vi "Origin_Export_7_27a_JW.vi"(6 "Input Conditions":T1, 7 "Analysis Array":string[][](array[string]), 8 "error in (no error)":errorcluster, 9 "Parameter Worksheet Name":string, 10 "Parameter Folder Script":string, 11 "Origin.IOApplication":refnum<k7>) -> (0 "error out":errorcluster, 2 "Origin.Worksheet":refnum<k7>, 3 "reference out":refnum<k7>)   [LabVIEW 2012]
panel:
  out "Dep Active Window":string
  out "Indep Unit":string
  out "Dep Unit":string
  out "Dep Used":string
  out "Indep Used":string
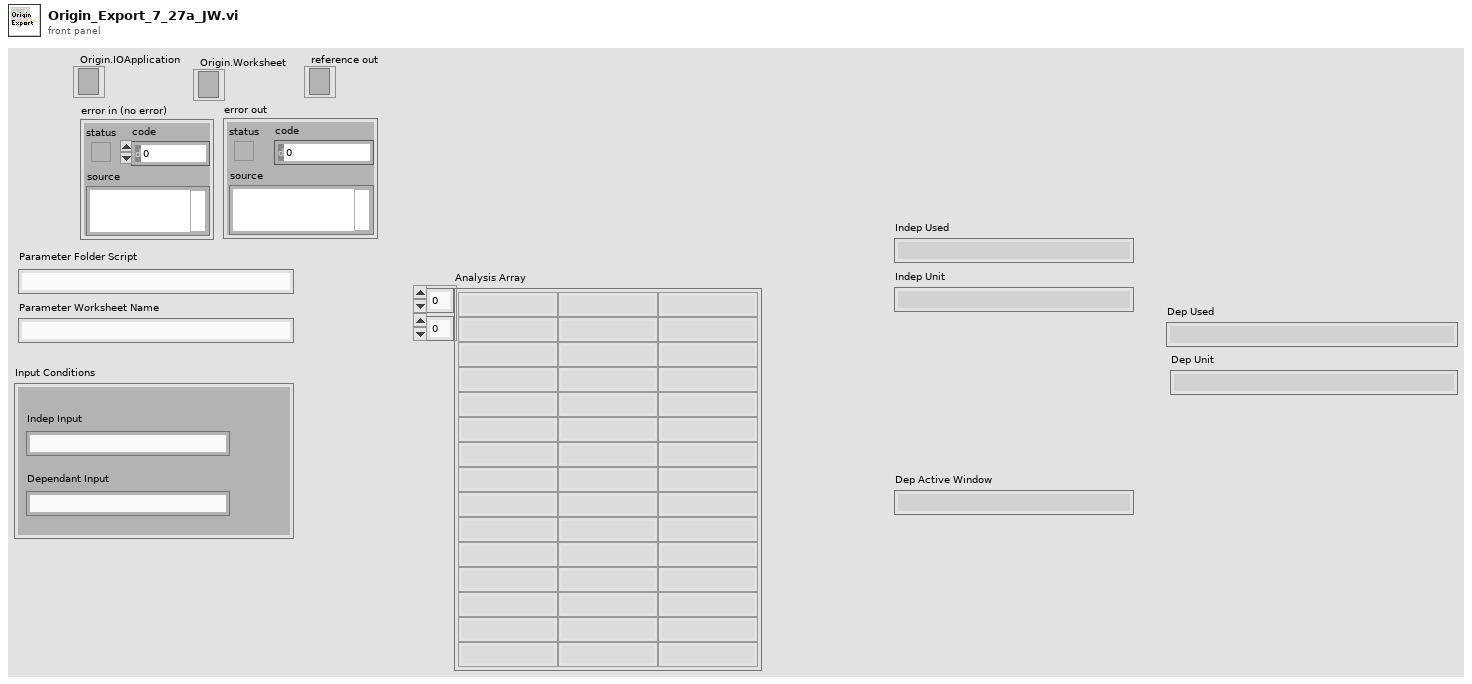
[diagram p1: front panel]
types:
  T1 = cluster{"Indep Input":string, "Dependant Input":string}
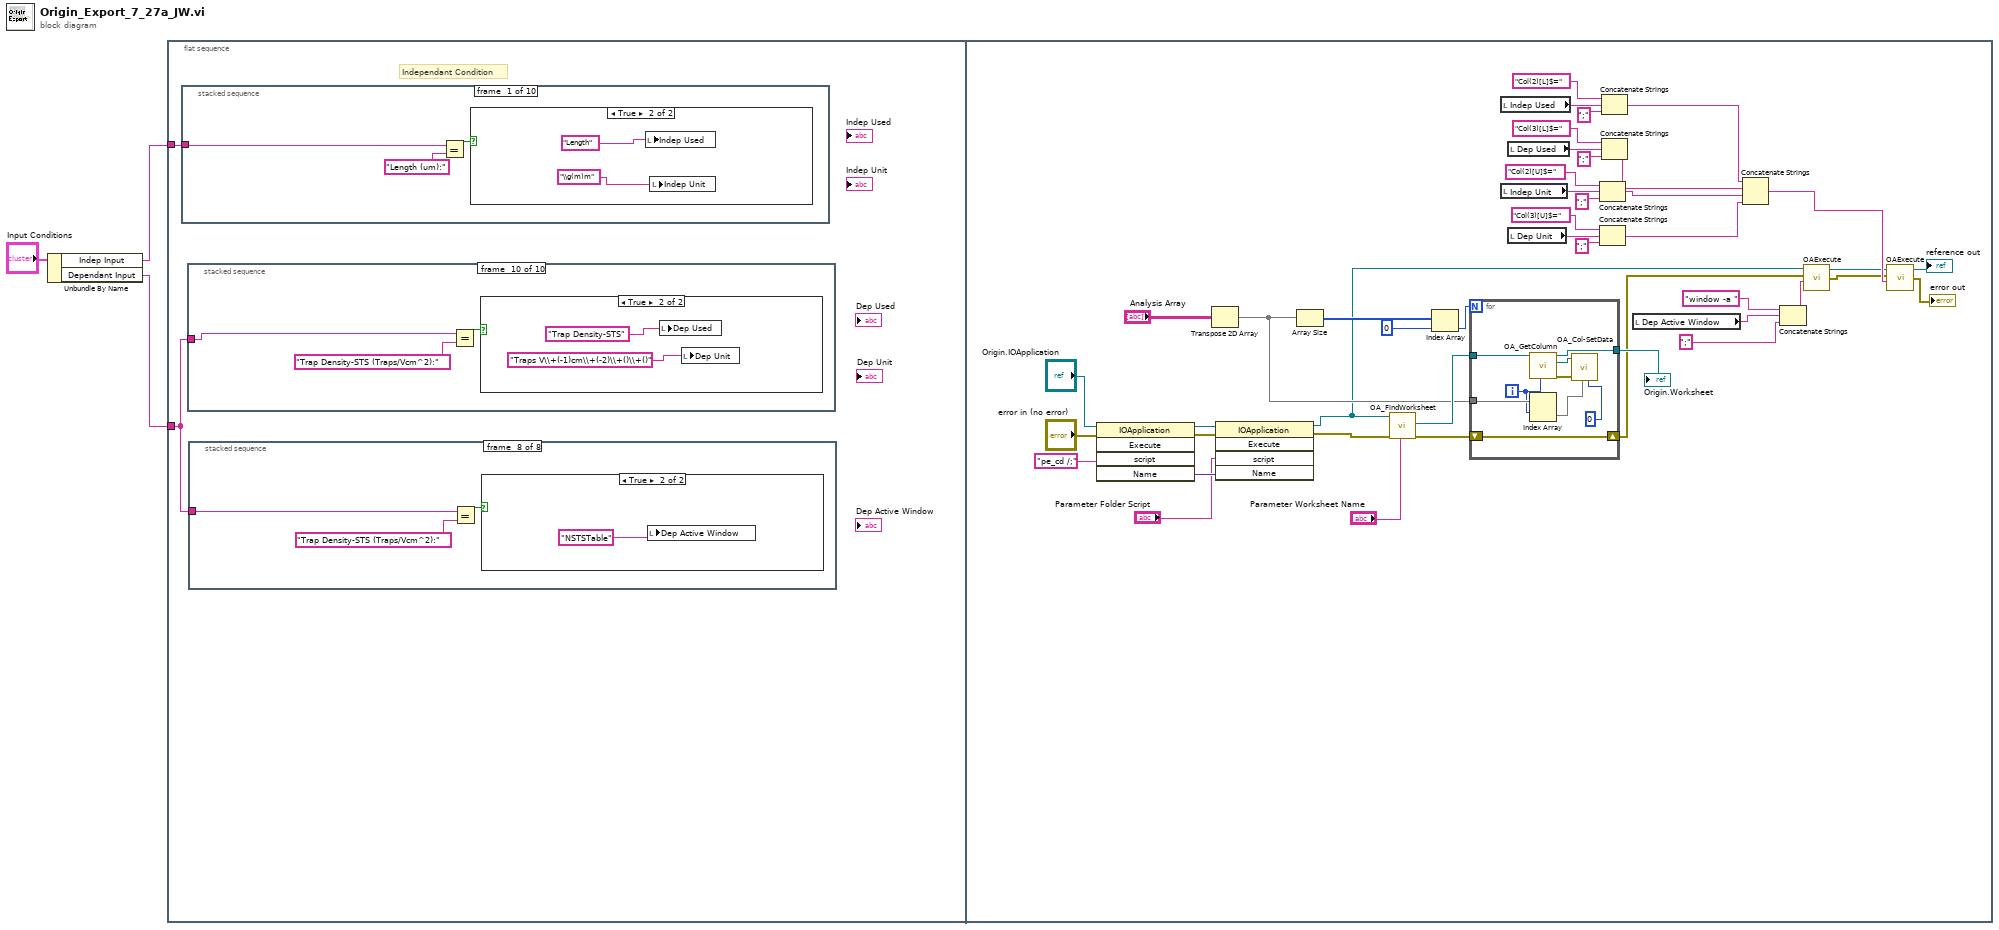
[diagram p0: block diagram]
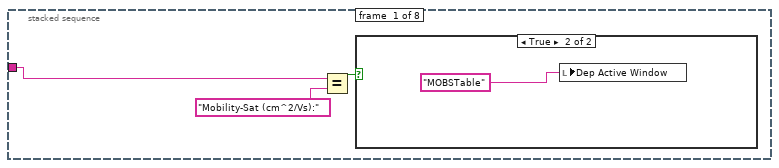
[diagram p2: hidden frame]
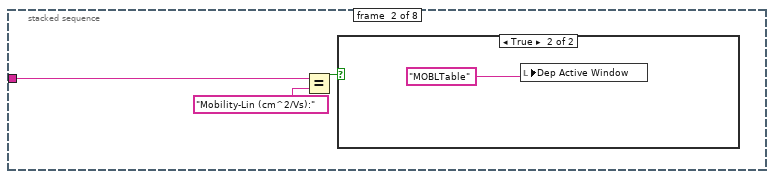
[diagram p4: hidden frame]
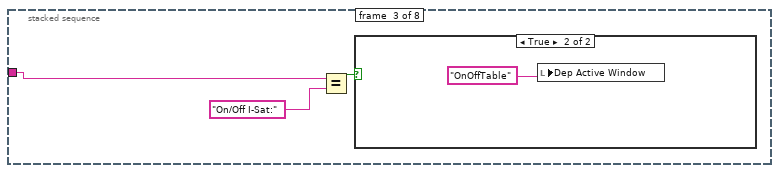
[diagram p6: hidden frame]
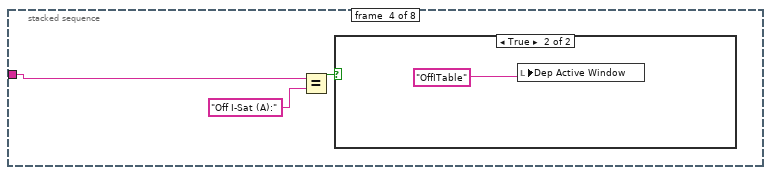
[diagram p8: hidden frame]
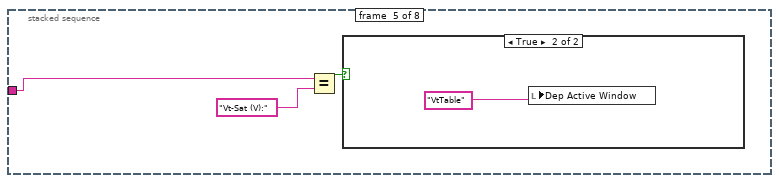
[diagram p10: hidden frame]
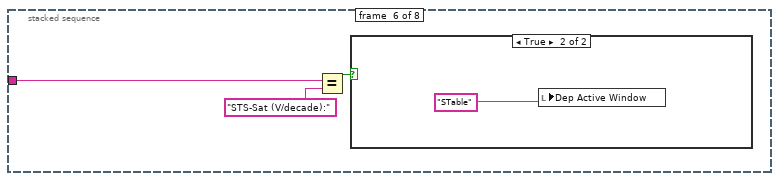
[diagram p12: hidden frame]
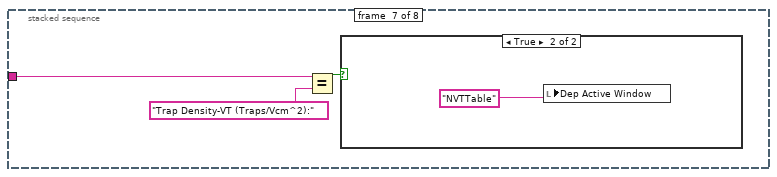
[diagram p14: hidden frame]
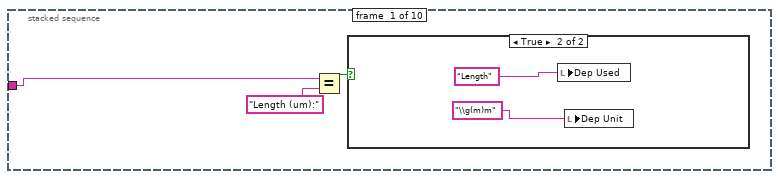
[diagram p17: hidden frame]
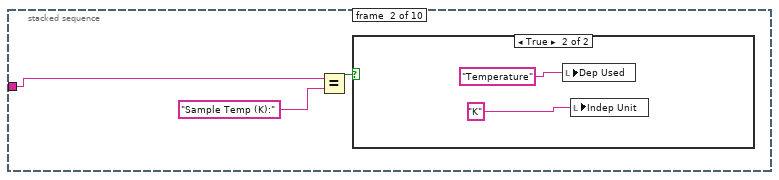
[diagram p19: hidden frame]
diagram:
  n1 = Unbundle By Name("Input Conditions") -> ("Indep Input"=w2:string, "Dependant Input"=w1:string)
  n2 = flat-sequence {
    tunnel: w2 -> [w5]
    tunnel: w1 -> [w4]
    frame #0 {
      # "Independant Condition"
      n3 = stacked-sequence {
        tunnel: w5 -> [w88 w93 w98 w103 w108 w113 w118 w123 w128 w133]
        frame #0 {
          n4 = Equal?(x=w88, y="Length (um):") -> (x = y?=w89:bool)
          n5 = case shown="True" w89 {
            frame False {
            }
            frame True {
              n6 = local write "Indep Used"("Length") -> ()
              n7 = local write "Indep Unit"("\\g(m)m") -> ()
            }
          }
        }
        frame #1 {
          n8 = Equal?(x=w93, y="Sample Temp (K):") -> (x = y?=w94:bool)
          n9 = case shown="True" w94 {
            frame False {
            }
            frame True {
              n10 = local write "Indep Used"("Temperature") -> ()
              n11 = local write "Indep Unit"("K") -> ()
            }
          }
        }
        frame #2 {
          n12 = Equal?(x=w98, y="Mobility-Sat (cm^2/Vs):") -> (x = y?=w99:bool)
          n13 = case shown="True" w99 {
            frame False {
            }
            frame True {
              n14 = local write "Indep Used"("Saturation Mobility") -> ()
              n15 = local write "Indep Unit"("cm\\+(2)V\\+(-1)s\\+(-1)") -> ()
            }
          }
        }
        frame #3 {
          n16 = Equal?(x=w103, y="Mobility-Lin (cm^2/Vs):") -> (x = y?=w104:bool)
          n17 = case shown="True" w104 {
            frame False {
            }
            frame True {
              n18 = local write "Indep Used"("Linear Mobility") -> ()
              n19 = local write "Indep Unit"("cm\\+(2)V\\+(-1)s\\+(-1)") -> ()
            }
          }
        }
        frame #4 {
          n20 = Equal?(x=w108, y="On/Off I-Sat:") -> (x = y?=w109:bool)
          n21 = case shown="True" w109 {
            frame False {
            }
            frame True {
              n22 = local write "Indep Used"("On/Off Current") -> ()
              n23 = local write "Indep Unit"("") -> ()
            }
          }
        }
        frame #5 {
          n24 = Equal?(x=w113, y="Off I-Sat (A):") -> (x = y?=w114:bool)
          n25 = case shown="True" w114 {
            frame False {
            }
            frame True {
              n26 = local write "Indep Used"("Off Current") -> ()
              n27 = local write "Indep Unit"("A") -> ()
            }
          }
        }
        frame #6 {
          n28 = Equal?(x=w118, y="Vt-Sat (V):") -> (x = y?=w119:bool)
          n29 = case shown="True" w119 {
            frame False {
            }
            frame True {
              n30 = local write "Indep Used"("Threshold Voltage") -> ()
              n31 = local write "Indep Unit"("V") -> ()
            }
          }
        }
        frame #7 {
          n32 = Equal?(x=w123, y="STS-Sat (V/decade):") -> (x = y?=w124:bool)
          n33 = case shown="True" w124 {
            frame False {
            }
            frame True {
              n34 = local write "Indep Used"("STS") -> ()
              n35 = local write "Indep Unit"("V dec\\+(-1)") -> ()
            }
          }
        }
        frame #8 {
          n36 = Equal?(x=w128, y="Trap Density-VT (Traps/Vcm^2):") -> (x = y?=w129:bool)
          n37 = case shown="True" w129 {
            frame False {
            }
            frame True {
              n38 = local write "Indep Used"("Trap Density-VT") -> ()
              n39 = local write "Indep Unit"("Traps V\\+(-1)cm\\+(-2)\\+()\\+()") -> ()
            }
          }
        }
        frame #9 {
          n40 = Equal?(x=w133, y="Trap Density-STS (Traps/Vcm^2):") -> (x = y?=w134:bool)
          n41 = case shown="True" w134 {
            frame False {
            }
            frame True {
              n42 = local write "Indep Used"("Trap Density-STS") -> ()
              n43 = local write "Indep Unit"("Traps V\\+(-1)cm\\+(-2)\\+()\\+()") -> ()
            }
          }
        }
      }
      n44 = stacked-sequence {
        tunnel: w4 -> [w38 w43 w48 w53 w58 w63 w68 w73 w78 w83]
        frame #0 {
          n45 = Equal?(x=w38, y="Length (um):") -> (x = y?=w39:bool)
          n46 = case shown="True" w39 {
            frame False {
            }
            frame True {
              n47 = local write "Dep Used"("Length") -> ()
              n48 = local write "Dep Unit"("\\g(m)m") -> ()
            }
          }
        }
        frame #1 {
          n49 = Equal?(x=w43, y="Sample Temp (K):") -> (x = y?=w44:bool)
          n50 = case shown="True" w44 {
            frame False {
            }
            frame True {
              n51 = local write "Dep Used"("Temperature") -> ()
              n52 = local write "Indep Unit"("K") -> ()
            }
          }
        }
        frame #2 {
          n53 = Equal?(x=w48, y="Mobility-Sat (cm^2/Vs):") -> (x = y?=w49:bool)
          n54 = case shown="True" w49 {
            frame False {
            }
            frame True {
              n55 = local write "Dep Used"("Saturation Mobility") -> ()
              n56 = local write "Dep Unit"("cm\\+(2)V\\+(-1)s\\+(-1)") -> ()
            }
          }
        }
        frame #3 {
          n57 = Equal?(x=w53, y="Mobility-Lin (cm^2/Vs):") -> (x = y?=w54:bool)
          n58 = case shown="True" w54 {
            frame False {
            }
            frame True {
              n59 = local write "Dep Used"("Linear Mobility") -> ()
              n60 = local write "Dep Unit"("cm\\+(2)V\\+(-1)s\\+(-1)") -> ()
            }
          }
        }
        frame #4 {
          n61 = Equal?(x=w58, y="On/Off I-Sat:") -> (x = y?=w59:bool)
          n62 = case shown="True" w59 {
            frame False {
            }
            frame True {
              n63 = local write "Dep Unit"("") -> ()
              n64 = local write "Dep Used"("On/Off Current") -> ()
            }
          }
        }
        frame #5 {
          n65 = Equal?(x=w63, y="Off I-Sat (A):") -> (x = y?=w64:bool)
          n66 = case shown="True" w64 {
            frame False {
            }
            frame True {
              n67 = local write "Dep Unit"("A") -> ()
              n68 = local write "Dep Used"("Off Current") -> ()
            }
          }
        }
        frame #6 {
          n69 = Equal?(x=w68, y="Vt-Sat (V):") -> (x = y?=w69:bool)
          n70 = case shown="True" w69 {
            frame False {
            }
            frame True {
              n71 = local write "Dep Used"("Threshold Voltage") -> ()
              n72 = local write "Dep Unit"("V") -> ()
            }
          }
        }
        frame #7 {
          n73 = Equal?(x=w73, y="STS-Sat (V/decade):") -> (x = y?=w74:bool)
          n74 = case shown="True" w74 {
            frame False {
            }
            frame True {
              n75 = local write "Dep Used"("STS") -> ()
              n76 = local write "Dep Unit"("V dec\\+(-1)") -> ()
            }
          }
        }
        frame #8 {
          n77 = Equal?(x=w78, y="Trap Density-VT (Traps/Vcm^2):") -> (x = y?=w79:bool)
          n78 = case shown="True" w79 {
            frame False {
            }
            frame True {
              n79 = local write "Dep Used"("Trap Density-VT") -> ()
              n80 = local write "Dep Unit"("Traps V\\+(-1)cm\\+(-2)\\+()\\+()") -> ()
            }
          }
        }
        frame #9 {
          n81 = Equal?(x=w83, y="Trap Density-STS (Traps/Vcm^2):") -> (x = y?=w84:bool)
          n82 = case shown="True" w84 {
            frame False {
            }
            frame True {
              n83 = local write "Dep Used"("Trap Density-STS") -> ()
              n84 = local write "Dep Unit"("Traps V\\+(-1)cm\\+(-2)\\+()\\+()") -> ()
            }
          }
        }
      }
      n85 = stacked-sequence {
        tunnel: w4 -> [w6 w10 w14 w18 w22 w26 w30 w34]
        frame #0 {
          n86 = Equal?(x=w6, y="Mobility-Sat (cm^2/Vs):") -> (x = y?=w7:bool)
          n87 = case shown="True" w7 {
            frame False {
            }
            frame True {
              n88 = local write "Dep Active Window"("MOBSTable") -> ()
            }
          }
        }
        frame #1 {
          n89 = Equal?(x=w10, y="Mobility-Lin (cm^2/Vs):") -> (x = y?=w11:bool)
          n90 = case shown="True" w11 {
            frame False {
            }
            frame True {
              n91 = local write "Dep Active Window"("MOBLTable") -> ()
            }
          }
        }
        frame #2 {
          n92 = Equal?(x=w14, y="On/Off I-Sat:") -> (x = y?=w15:bool)
          n93 = case shown="True" w15 {
            frame False {
            }
            frame True {
              n94 = local write "Dep Active Window"("OnOffTable") -> ()
            }
          }
        }
        frame #3 {
          n95 = Equal?(x=w18, y="Off I-Sat (A):") -> (x = y?=w19:bool)
          n96 = case shown="True" w19 {
            frame False {
            }
            frame True {
              n97 = local write "Dep Active Window"("OffITable") -> ()
            }
          }
        }
        frame #4 {
          n98 = Equal?(x=w22, y="Vt-Sat (V):") -> (x = y?=w23:bool)
          n99 = case shown="True" w23 {
            frame False {
            }
            frame True {
              n100 = local write "Dep Active Window"("VtTable") -> ()
            }
          }
        }
        frame #5 {
          n101 = Equal?(x=w26, y="STS-Sat (V/decade):") -> (x = y?=w27:bool)
          n102 = case shown="True" w27 {
            frame False {
            }
            frame True {
              n103 = local write "Dep Active Window"("STable") -> ()
            }
          }
        }
        frame #6 {
          n104 = Equal?(x=w30, y="Trap Density-VT (Traps/Vcm^2):") -> (x = y?=w31:bool)
          n105 = case shown="True" w31 {
            frame False {
            }
            frame True {
              n106 = local write "Dep Active Window"("NVTTable") -> ()
            }
          }
        }
        frame #7 {
          n107 = Equal?(x=w34, y="Trap Density-STS (Traps/Vcm^2):") -> (x = y?=w35:bool)
          n108 = case shown="True" w35 {
            frame False {
            }
            frame True {
              n109 = local write "Dep Active Window"("NSTSTable") -> ()
            }
          }
        }
      }
    }
    frame #1 {
      n110 = invoke class="IOApplication" method="Execute"(reference="Origin.IOApplication", error in="error in (no error)", "script"="pe_cd /;") -> (reference out=w180:refnum<k7>, error out=w179:errorcluster, "Name"=w178:variant)  [unwired: 2 in, 2 out]
      n111 = Transpose 2D Array(2D array="Analysis Array") -> (transposed array=w171:string[][])
      n112 = invoke class="IOApplication" method="Execute"(reference=w180, error in=w179, "script"="Parameter Folder Script", "Name"=w178) -> (reference out=w145:refnum<k7>, error out=w167:errorcluster)  [unwired: 1 in, 3 out]
      n113 = Array Size(array=w171) -> (size(s)=w175:i32[])
      n114 = call "OA_FindWorksheet.vi"("Name"="Parameter Worksheet Name", "error in (no error)"=w167, "Origin.IOApplication"=w145) -> ("error out"=w176:errorcluster, "Origin.Worksheet"=w177:refnum<k7>)  [unwired: 6 in, 1 out]
      n115 = Index Array(array=w175, index=0) -> (element=w174:i32)
      n116 = for {
        N: w174 -> [_]
        tunnel: w177 -> [w190]
        tunnel: w171 -> [w189]
        tunnel: [w188] -> w172
        shift-right: [w184] -> w147
        shift-left: w176 -> [w184]
        i -> [w183]
        n117 = call "OA_GetColumn.vi"("Column Name/Index"=w183, "Origin.Worksheet"=w190) -> ("error out"=w186:errorcluster, "Origin.Column"=w187:refnum<k7>, "Origin.Worksheet"=w188:refnum<k7>)  [unwired: 7 in]
        n118 = Index Array(array=w189, index (row)=w183) -> (element=w185:string[])  [unwired: 1 in]
        n119 = call "OA_Col-SetData.vi"("Origin.Column"=w187, "error in (no error)"=w186, "data"=w185, "nOffset"=0) -> ()  [unwired: 3 in, 3 out]
      }
      "Origin.Worksheet" <- w172
      n120 = local read "Indep Used"() -> (w151:string)
      n121 = local read "Indep Unit"() -> (w156:string)
      n122 = local read "Dep Used"() -> (w152:string)
      n123 = local read "Dep Unit"() -> (w157:string)
      n124 = Concatenate Strings("Col(2)[U]$=", w156, ";") -> (w154:string)
      n125 = Concatenate Strings("Col(3)[U]$=", w157, ";") -> (w153:string)
      n126 = Concatenate Strings("Col(2)[L]$=", w151, ";") -> (w148:string)
      n127 = Concatenate Strings("Col(3)[L]$=", w152, ";") -> (w150:string)
      n128 = local read "Dep Active Window"() -> (w142:string)
      n129 = Concatenate Strings(w148, w150, w154, w153) -> (w149:string)
      n130 = Concatenate Strings("window -a ", w142, ";") -> (w140:string)
      n131 = call "OAExecute.vi"("script"=w140, "Error IO"=w147, "Origin.IOApplication"=w145) -> ("Error IO Out"=w146:errorcluster, "Origin.IOApplication"=w144:refnum<k7>)  [unwired: 1 in, 1 out]
      n132 = call "OAExecute.vi"("script"=w149, "Error IO"=w146, "Origin.IOApplication"=w144) -> ("Error IO Out"=→"error out":errorcluster, "Origin.IOApplication"=→"reference out":refnum<k7>)  [unwired: 1 in, 1 out]
    }
  }
